vi "Set DataType.vi"(8 "error in":errorcluster, 10 "Value":refnum<class "Value.lvclass">, 11 "Object Type in":refnum<class "Object Type Base.lvclass">) -> (0 "error out":errorcluster, 3 "Object Type out":refnum<class "Object Type Base.lvclass">)   [LabVIEW 2024, in "Electronic Datasheet.lvlib" / "Object Type Base.lvclass"]
uses:
  Object Type Base.lvclass
  Object Type Base.lvclass/Object Type Base.ctl
  Value/Value.lvclass
  Data Type.ctl
  Electronic Datasheet.lvlib
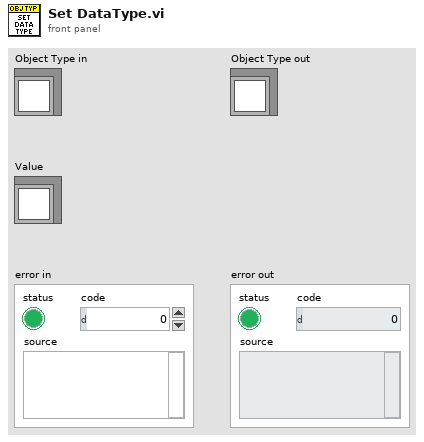
[diagram p1: front panel]
types:
  T1 = typedef "Electronic Datasheet.lvlib/Data Type.ctl" = u16
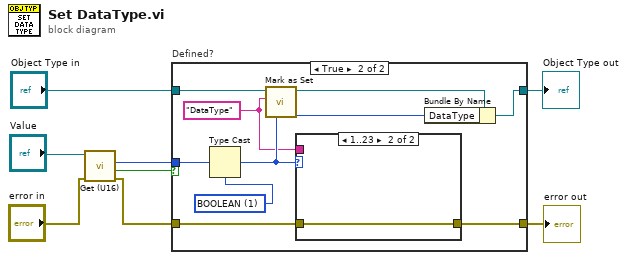
[diagram p0: block diagram]
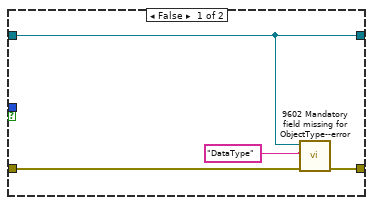
[diagram p2: hidden frame]
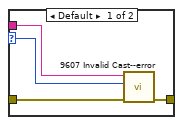
[diagram p3: hidden frame]
diagram:
  n1 = call "Get (U16).vi"("error in"="error in", "Value in"="Value") -> ("error out"=w1:errorcluster, "Defined?"=w5:bool, "Value"=w4:u16)  [unwired: 6 in, 1 out]
  n2 = case "Defined?" shown="True" w5 {
    tunnel: "Object Type in" -> [w9 w21]
    tunnel: [w9 w20] -> w7
    tunnel: w4 -> [_ w18]
    tunnel: w1 -> [w12 w15]
    tunnel: [w11 w14] -> w3
    frame False {
      n3 = call "9602 Mandatory field missing for ObjectType--error.vi"("error in"=w12, "Field Name"="DataType" ("error message (\"\")"), "Object Type Base"=w9) -> ("error out"=w11:errorcluster)  [unwired: 8 in]
    }
    frame True {
      w17 = T1 1 items=["BOOLEAN"=1, "INTEGER8"=2, "INTEGER16"=3, "INTEGER32"=4, "UNSIGNED8"=5, "UNSIGNED16"=6, "UNSIGNED32"=7, "REAL32"=8, "VISIBLE_STRING"=9, "OCTET_STRING"=10, "UNICODE_STRING"=11, "TIME_OF_DAY"=12, "TIME_DIFFERENCE"=13, "RESERVED1"=14, "DOMAIN"=15, "INTEGER24"=16, "REAL64"=17, "INTEGER40"=18, "INTEGER48"=19, "INTEGER56"=20, "INTEGER64"=21, "UNSIGNED24"=22, "RESERVED2"=23, "UNSIGNED40"=24, "UNSIGNED48"=25, "UNSIGNED56"=26, "UNSIGNED64"=27, "RESERVED3"=28, "RESERVED4"=29, "RESERVED5"=30, "RESERVED6"=31, "PDO_COMMUNICATION_PARAMETER"=32, "PDO_MAPPING"=33, "SDO_PARAMETER"=34, "IDENTITY"=35, "RESERVED7"=36] ("DataType")
      w13 = "DataType" ("Field name")
      n4 = Type Cast(type=w17, x=w18) -> (*(type *) &x=w16:T1)
      n5 = call "Mark as Set.vi"("Field name"=w13, "Object Type in"=w21) -> ("Object Type out"=w19:refnum<class "Object Type Base.lvclass">)  [unwired: 9 in]
      n6 = case shown="1..23" w16 {
        selector: w16 -> [w22 _]
        tunnel: w15 -> [w25 w26]
        tunnel: [w24 w26] -> w14
        tunnel: w13 -> [w23 _]
        frame Default {
          n7 = call "9607 Invalid Cast--error.vi"("error in"=w25, "Value"=w22, "Type"=w23) -> ("error out"=w24:errorcluster)  [unwired: 8 in]
        }
        frame 1..35 {
        }
      }
      n8 = Bundle By Name(cluster=w19, "DataType"=w16) -> (w20:refnum<class "Object Type Base.lvclass">)
    }
  }
  "Object Type out" <- w7
  "error out" <- w3
